vi "Data Trends Control.vi"(8 "error in (no error)":errorcluster, 10 "Metadata in":string[][](array[string]), 11 "Message Queues In":T1) -> (0 "error out":errorcluster)   [LabVIEW 2014, in "Data Trends.lvlib"]
uses:
  Data Trends.lvlib
  Support/MeasurementControl Message Queue Folder/All Message Queues.ctl
  Support/MeasurementControl Message Queue Folder/Message Cluster.ctl
  Support/MeasurementControl Message Queue Folder/MeasurementControl Message Queue.lvlib
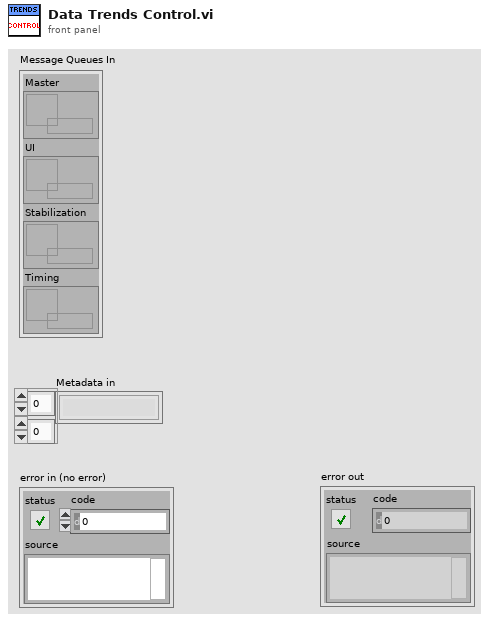
[diagram p1: front panel]
types:
  T1 = typedef "MeasurementControl Message Queue.lvlib/All Message Queues.ctl" = cluster{"Master":refnum<queue>, "UI":refnum<queue>, "Stabilization":refnum<queue>, "Timing":refnum<queue>}
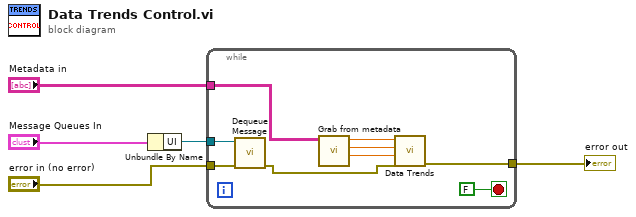
[diagram p0: block diagram]
diagram:
  n1 = Unbundle By Name("Message Queues In") -> ("UI"=w1:refnum<queue>)
  n2 = while {
    tunnel: "error in (no error)" -> [w8]
    tunnel: [w11] -> w4
    tunnel: "Metadata in" -> [w7]
    tunnel: w1 -> [w6]
    stop <- FALSE stop-if-true
    n3 = call "Dequeue Message.vi"("error in (no error)"=w8, "Message Queue"=w6) -> ("error out"=w9:errorcluster)  [unwired: 6 in, 3 out]
    n4 = call "Grab from metadata.vi"("Metadata in"=w7) -> ("hours"=w12:dbl, "sample"=w13:dbl, "model"=w14:dbl)  [unwired: 8 in]
    n5 = call "Data Trends.vi"("error in (no error)"=w9, "Hours"=w12, "Sample"=w13, "Model"=w14) -> ("error out"=w11:errorcluster)  [unwired: 3 in, 4 out]
  }
  "error out" <- w4
